vi "ReadMatrixSub.vi"(8 "error in (no error)":errorcluster) -> (0 "error out":errorcluster, 2 "Array 2":string[](array[string]), 3 "Array":bool[][](array[boolean]))   [LabVIEW 2017]
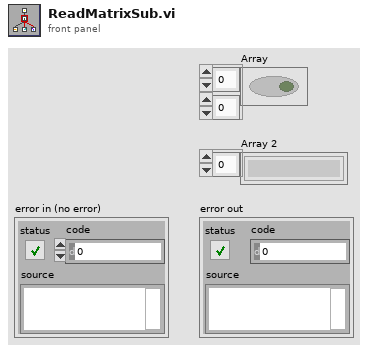
[diagram p1: front panel]
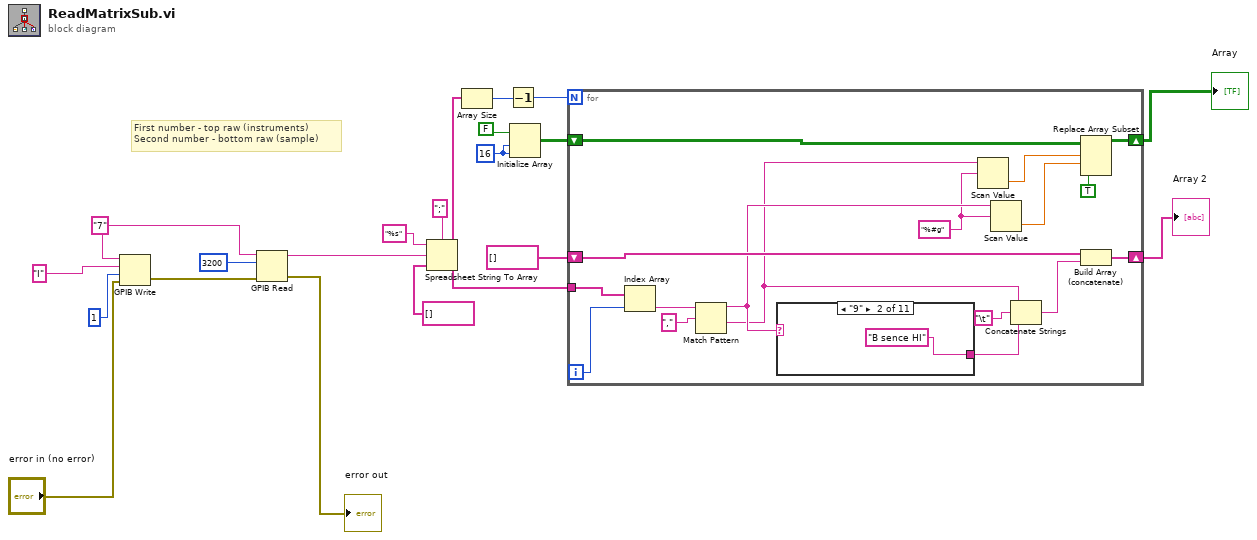
[diagram p0: block diagram]
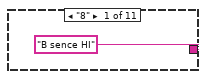
[diagram p2: hidden frame]
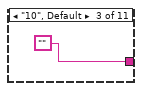
[diagram p3: hidden frame]
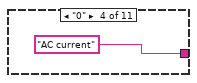
[diagram p4: hidden frame]
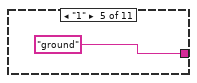
[diagram p5: hidden frame]
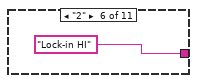
[diagram p6: hidden frame]
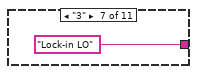
[diagram p7: hidden frame]
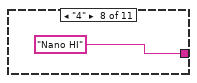
[diagram p8: hidden frame]
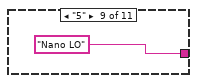
[diagram p9: hidden frame]
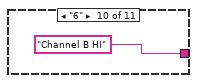
[diagram p10: hidden frame]
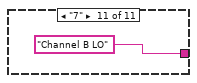
[diagram p11: hidden frame]
diagram:
  w18 = 16
  w5 = "7"
  # "First number - top raw (instruments)\nSecond number - bottom raw (sample)"
  n1 = GPIB Write(0:w5, 1:"I", 2:1, 3:"error in (no error)") -> (6:w1:errorcluster)  [unwired: 1 in, 1 out]
  n2 = GPIB Read(0:w5, 1:3200, 3:w1) -> (5:w8:string, 7:→"error out":errorcluster)  [unwired: 2 in, 1 out]
  n3 = Spreadsheet String To Array(delimiter (Tab)=";", format string="%s", spreadsheet string=w8, array type (2D Dbl)=string[] []) -> (array=w11:string[])
  n4 = Array Size(array=w11) -> (size(s)=w12:i32)
  n5 = Decrement(x=w12) -> (x-1=w13:i32)
  n6 = Initialize Array(FALSE, w18, w18) -> (w19:bool[][])
  n7 = for {
    N: w13 -> [_]
    tunnel: w11 -> [w37]
    shift-right: [w31] -> w15
    shift-left: string[] [] -> [w32]
    shift-right: [w27] -> w20
    shift-left: w19 -> [w28]
    i -> [w36]
    w21 = "%#g"
    n8 = Index Array(array=w37, index=w36) -> (element=w34:string)
    n9 = Match Pattern(string=w34, regular expression=",") -> (before substring=w26:string, after substring=w25:string)  [unwired: 1 in, 2 out]
    n10 = case shown="\"9\"" w26 {
      tunnel: ["B sence HI" "B sence HI" "" "AC current" "ground" "Lock-in HI" "Lock-in LO" "Nano HI" "Nano LO" "Channel B HI" "Channel B LO"] -> w30
      frame "8" {
      }
      frame "9" {
      }
      frame "10", Default {
      }
      frame "0" {
      }
      frame "1" {
      }
      frame "2" {
      }
      frame "3" {
      }
      frame "4" {
      }
      frame "5" {
      }
      frame "6" {
      }
      frame "7" {
      }
    }
    n11 = Scan Value(string=w25, format string=w21) -> (value=w24:dbl)  [unwired: 1 in, 1 out]
    n12 = Scan Value(string=w26, format string=w21) -> (value=w22:dbl)  [unwired: 1 in, 1 out]
    n13 = Concatenate Strings(w25, "\t", w30) -> (w33:string)
    n14 = Replace Array Subset(array=w28, new element=TRUE, index (row)=w24, index (col)=w22) -> (w27:bool[][])
    n15 = Build Array (concatenate)(w32, w33) -> (w31:string[])
  }
  "Array" <- w20
  "Array 2" <- w15
